vi "Interface tset.vi"() -> ()   [LabVIEW 2011]
uses:
  Criteria types.ctl
  Single criteria cluster.ctl
  Boolean operation.ctl
  Sequence steps config..ctl
  X-cont criteria/Criteria control.xctl
  Sequence step GUI.ctl
  X-cont Action select/Action select.xctl
  <vilib>/Utility/config.llb/NI_LVConfig.lvlib
panel:
  in  "Read":bool
  in  "Sequewnce jname":string="test"
  in  "Lagr":bool
  in  "Get":bool
  in  "Index":i32
  out "Array":string[](array[string])
  in  "Add":bool
  in  "Criteria 2":cluster{"Criteria":T1}(xcontrol)
  in  "Action select":cluster{"Action index":i32, "Data":dbl}(xcontrol)
  in  "Cluster 3":cluster{"Cluster 2":T3}
  out "Sequence step config":T5
  in  "Cluster":T3
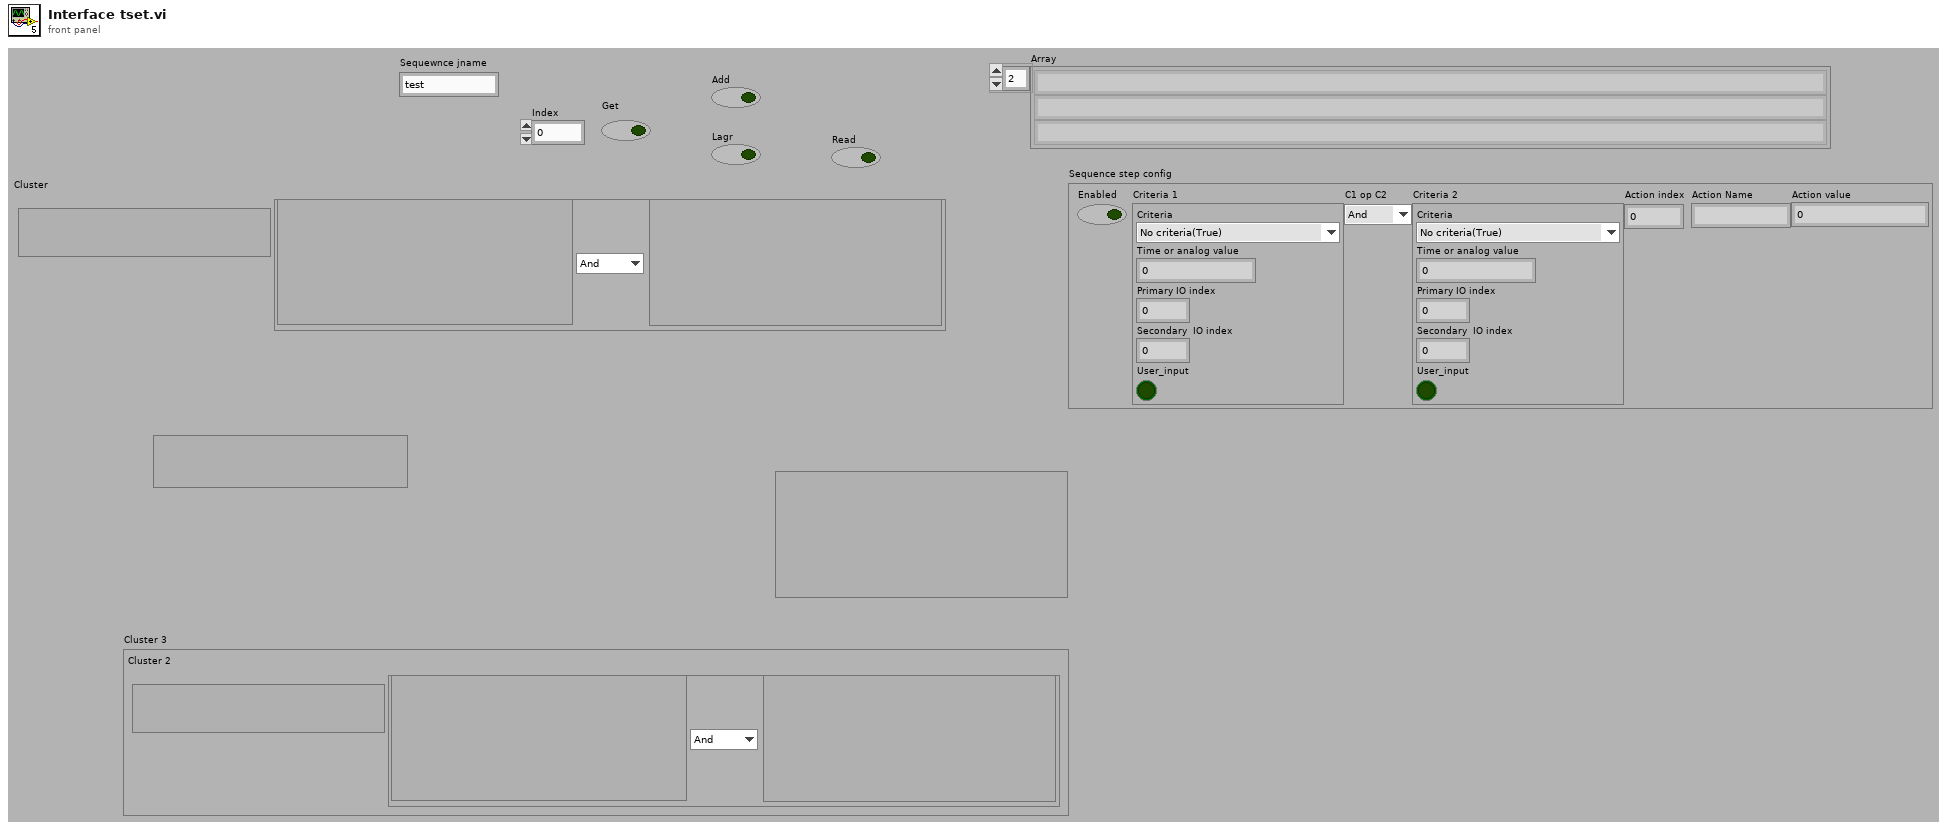
[diagram p1: front panel]
types:
  T1 = typedef "Single criteria cluster.ctl" = cluster{"Criteria":T2, "Time or analog value":dbl, "Primary IO index":i32, "Secondary  IO index":i32, "User_input":bool}
  T2 = typedef "Criteria types.ctl" = enum16{"No criteria(True)", "Time(s)", "Analog IO over", "Analog IO over or equal", "Analog IO under", "Analog IO under or equal", "Analog IO 1 minus Analog IO 2 over", "Digital IO True", "Digital IO False", "Operator approval"}
  T3 = typedef "Sequence step GUI.ctl" = cluster{"Action select":cluster{"Action index":i32, "Data":dbl}, "Criteria 1":cluster{"Criteria":T1}, "C1 op C2":T4, "Criteria 2":cluster{"Criteria":T1}}
  T4 = typedef "Boolean operation.ctl" = enum16{"And", "Or", "Xor", "Nand", "Nor", "Nxor", "Implies"}
  T5 = typedef "Sequence steps config..ctl" = cluster{"Enabled":bool, "Criteria 1":T1, "C1 op C2":T4, "Criteria 2":T1, "Action index":i32, "Action Name":string, "Action value":dbl}
  T6 = typedef "Action colleciton cluster.ctl" = cluster{"common":T7, "Action type":T9, "General command":T10, "PCP command":T11, "Tool command":T12}
  T7 = typedef "Action common elements.ctl" = cluster{"Name":string, "Adjuster type":T8, "Adjuster double default value":dbl}
  T8 = typedef "Action adjuster type.ctl" = enum16{"Non", "Double"}
  T9 = typedef "Action type.ctl" = enum16{"General", "PCP command", "Tool command"}
  T10 = typedef "General command list.ctl" = enum16{"No action"}
  T11 = typedef "PCP High Level Commands.ctl" = enum16{"HVPSU HV ON", "HVPSU HV OFF", "PCP PC", "PCP Local", "Update Motor Voltage", "Update Cable Resistance", "Final Motor Voltage", "Final Resistance"}
  T12 = typedef "Tool specific commands.ctl" = enum16{"controller relay 1 on", "controller relay 1 off", "controller relay 2 on", "controller relay 2 off", "Solonoid 1 (master) on", "Solonoid 1 (master) off", "Solonoid 2 (Stroker) on", "Solonoid 2 (Stroker) off", "Solonoid 3 (Anchor) on", "Solonoid 3 (Anchor) off", "Controller relay 1 & 2 on", "Controller relay 1 & 2 off", "Controller relay 1 on, 2 off", "Controller relay 1 off, 2 on", "STROKER tool: Stop Force Mon", "High-G Stop", "High-G Get data", "High-G Stop Get data", "STROKER tool: Stroke out", "STROKER tool: Stroke in", "STROKER tool: Stroke stop", "STROKER tool: Stroke go to", "STROKER tool: Stop Homing", "STROKER tool: Start Force Mon dir in", "STROKER tool: Start Force Mon dir out", "Controller STOP"}
  T13 = typedef "Fixed Analog Channel Definition.ctl" = cluster{"ID":u16, "Name":string, "Quantity":T14, "Unit":string, "Maximum upd":T15, "Comment":string, "Help file Name":string, "Help file Section ":string, "Category":T16, "User adjustable Scaling":bool, "Default Scaling":T17, "In use":bool, "Default Unit":i32}
  T14 = typedef "Quantity enum.ctl" = enum16{"Acceleration", "Angle", "Current", "Force", "Distance", "Pressure", "Resistance", "Rotational Speed", "Speed", "Temperature", "Tension", "Torque", "Voltage", "Weight"}
  T15 = typedef "Update frequensies.ctl" = enum16{"2 Hz", "1 Hz", "0.1 Hz"}
  T16 = typedef "Channel catagory Enum.ctl" = enum16{"No Category", "Power", "Temperature", "Pressure"}
  T17 = typedef "Scaling.ctl" = cluster{"Gain":dbl, "Offset":dbl}
  T18 = typedef "Fixed Digital Channel Definition.ctl" = cluster{"ID":u16, "Name":string, "NA Text":string, "Off Text":string, "On Text":string, "Maximum upd":T15, "Comment":string, "Help file Name":string, "Help file Section ":string, "Catagory":T16, "In use":bool}
  T19 = typedef "NI_LVConfig.lvlib/Config Data RefNum.ctl" = refnum<k1>
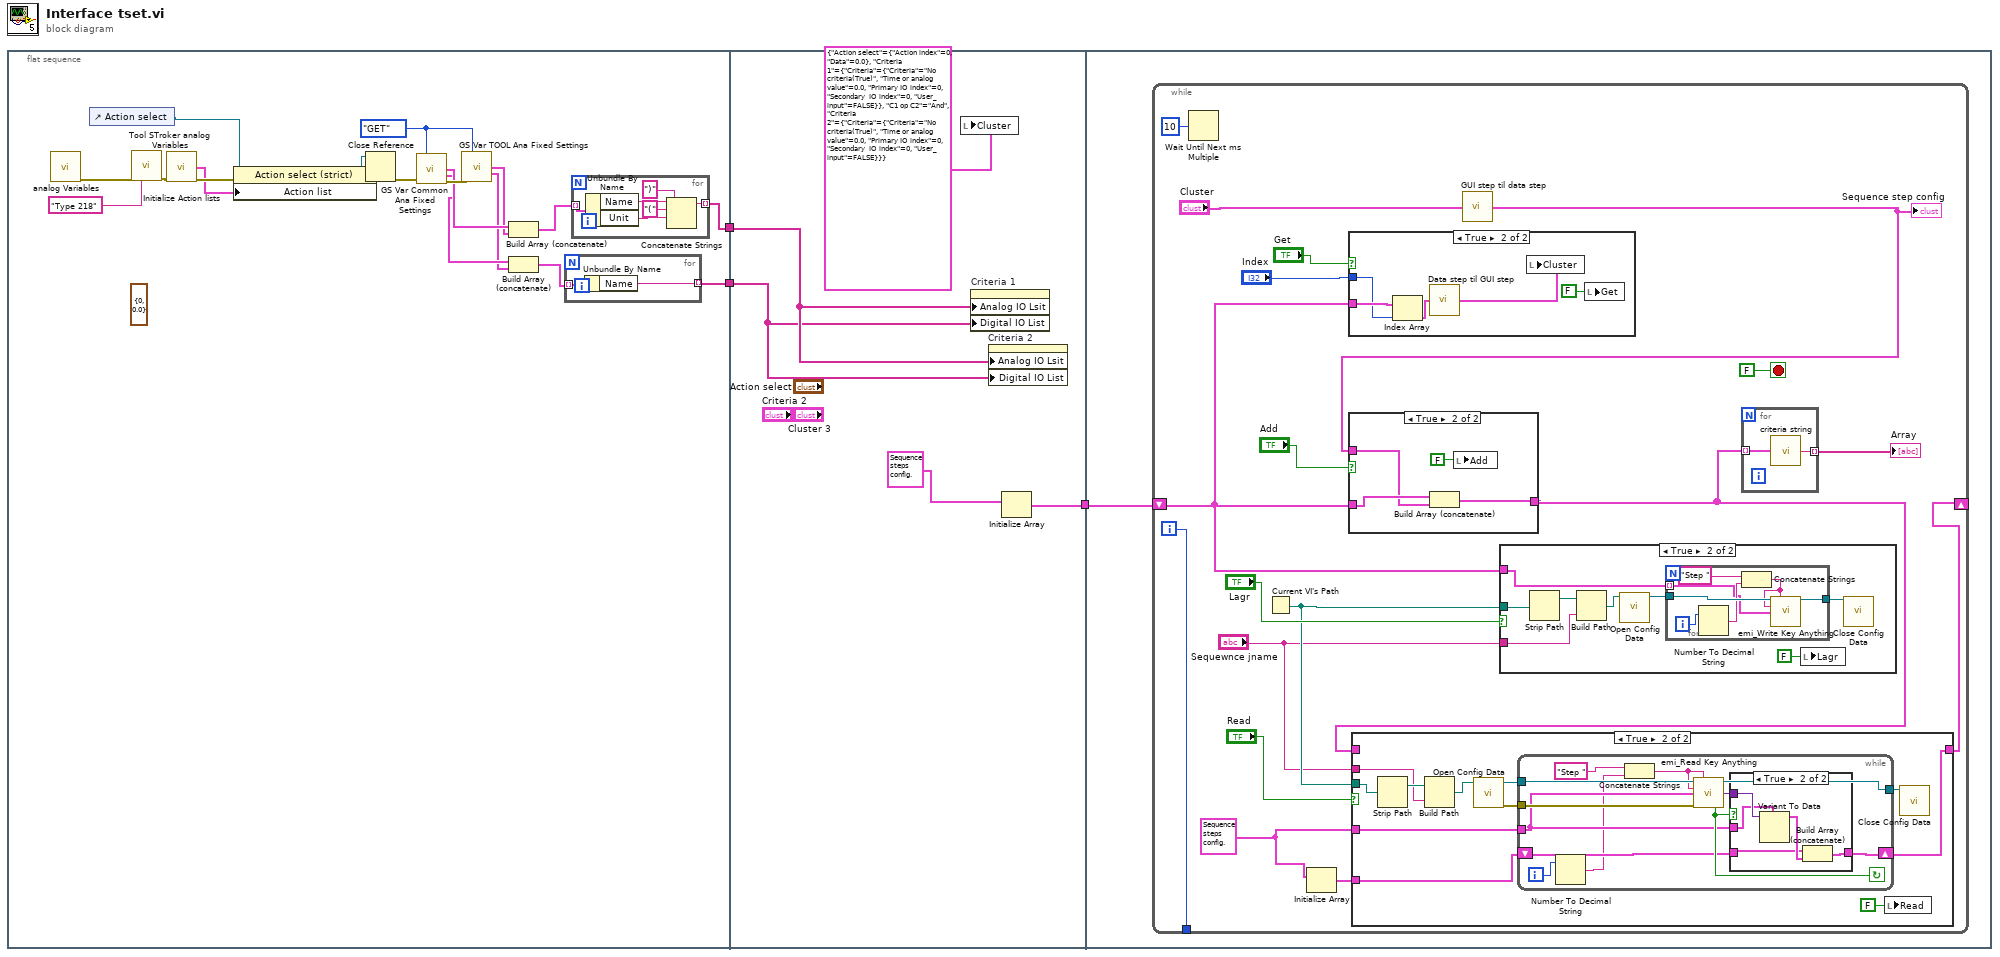
[diagram p0: block diagram]
diagram:
  n1 = flat-sequence {
    tunnel: [w7] -> w3
    tunnel: [w6] -> w2
    tunnel: w3 -> [w35]
    tunnel: w2 -> [w34]
    tunnel: [w31] -> w1
    tunnel: w1 -> [w36]
    frame #0 {
      (unwired) cluster{"Action index":i32, "Data":dbl} {"Action index"=0, "Data"=0.0} ("Action select")
      w14 = enum16{"GET", "SET"}."GET" ("Action(GET)")
      n2 = call "analog Variables.vi"() -> ("error out"=w19:errorcluster)  [unwired: 15 in]
      n3 = control-ref of="Action select"() -> (w5:refnum<vi>)
      n4 = call "Tool STroker analog Variables.vi"("error in (no error)"=w19, "Tool folder name"="Type 218") -> ("error out"=w18:errorcluster)  [unwired: 13 in]
      n5 = call "Initialize Action lists.vi"("error in (no error)"=w18) -> ("Actions"=w4:T6[], "error out"=w20:errorcluster)  [unwired: 12 in, 1 out]
      n6 = property class="Action select (strict)"(reference=w5, error in=w20, "Action list"=w4) -> (reference out=w22:refnum<vi>, error out=w21:errorcluster)
      n7 = Close Reference(reference=w22, error in (no error)=w21) -> (error out=w16:errorcluster)
      n8 = call "GS Var Common Ana Fixed Settings.vi"("Action(GET)"=w14, "error in (no error)"=w16) -> ("Common Analog Var Fixed out"=w13:T13[], "Common Digital var Fixed"=w11:T18[], "error out"=w15:errorcluster)  [unwired: 11 in]
      n9 = call "GS Var TOOL Ana Fixed Settings.vi"("Action(GET)"=w14, "error in (no error)"=w15) -> ("Tool Analog var Fixed out"=w12:T13[], "Tool Digital Var Fixed out"=w10:T18[])  [unwired: 11 in, 1 out]
      n10 = Build Array (concatenate)(w13, w12) -> (w9:T13[])
      n11 = Build Array (concatenate)(w11, w10) -> (w8:T18[])
      n12 = for {
        tunnel: w8 -> [w24] mode=indexing
        tunnel: [w23] -> w6 mode=indexing
        n13 = Unbundle By Name(w24) -> ("Name"=w23:string)
      }
      n14 = for {
        tunnel: w9 -> [w30] mode=indexing
        tunnel: [w28] -> w7 mode=indexing
        n15 = Unbundle By Name(w30) -> ("Name"=w29:string, "Unit"=w27:string)
        n16 = Concatenate Strings(w29, "(" ("string"), w27, ")" ("string")) -> (w28:string)
      }
    }
    frame #1 {
      n17 = local write "Cluster"(T3 {"Action select"={"Action index"=0, "Data"=0.0}, "Criteria 1"={"Criteria"={"Criteria"=enum."No criteria(True)", "Time or analog value"=0.0, "Primary IO index"=0, "Secondary  IO index"=0, "User_input"=FALSE}}, "C1 op C2"=enum."And", "Criteria 2"={"Criteria"={"Criteria"=enum."No criteria(True)", "Time or analog value"=0.0, "Primary IO index"=0, "Secondary  IO index"=0, "User_input"=FALSE}}} ("Cluster")) -> ()
      n18 = property on="Criteria 1" class="Criteria control (strict)"("Analog IO Lsit"=w35, "Digital IO List"=w34) -> ()  [unwired: 2 in, 2 out]
      n19 = property on="Criteria 2" class="Criteria control (strict)"("Analog IO Lsit"=w35, "Digital IO List"=w34) -> ()  [unwired: 2 in, 2 out]
      n20 = Initialize Array(T5 {"Enabled"=FALSE, "Criteria 1"={"Criteria"=enum."No criteria(True)", "Time or analog value"=0.0, "Primary IO index"=0, "Secondary  IO index"=0, "User_input"=FALSE}, "C1 op C2"=enum."And", "Criteria 2"={"Criteria"=enum."No criteria(True)", "Time or analog value"=0.0, "Primary IO index"=0, "Secondary  IO index"=0, "User_input"=FALSE}, "Action index"=0, "Action Name"="", "Action value"=0.0} ("Sequence step config")) -> (w31:T5[])  [unwired: 1 in]
    }
    frame #2 {
      n21 = while {
        shift-right: [w37] -> _
        shift-left: w36 -> [w45]
        tunnel: [w46] -> _
        i -> [w46]
        stop <- FALSE stop-if-true
        w40 = T5 {"Enabled"=FALSE, "Criteria 1"={"Criteria"=enum."No criteria(True)", "Time or analog value"=0.0, "Primary IO index"=0, "Secondary  IO index"=0, "User_input"=FALSE}, "C1 op C2"=enum."And", "Criteria 2"={"Criteria"=enum."No criteria(True)", "Time or analog value"=0.0, "Primary IO index"=0, "Secondary  IO index"=0, "User_input"=FALSE}, "Action index"=0, "Action Name"="", "Action value"=0.0} ("data step cluster")
        n22 = Wait Until Next ms Multiple(millisecond multiple=u32 10) -> ()  [unwired: 1 out]
        n23 = Current VI's Path() -> (path=w42:path)
        n24 = Initialize Array(w40) -> (w39:T5[])  [unwired: 1 in]
        n25 = case shown="True" "Get" {
          tunnel: "Index" -> [_ w102]
          tunnel: w45 -> [_ w103]
          frame False {
          }
          frame True {
            n26 = Index Array(array=w103, index=w102) -> (element=w101:T5)
            n27 = call "Data step til GUI step.vi"("data step cluster"=w101) -> ("GUI step clluster"=w100:T3)  [unwired: 13 in, 1 out]
            n28 = local write "Cluster"(w100) -> ()
            n29 = local write "Get"(FALSE ("Get")) -> ()
          }
        }
        n30 = call "GUI step til data step.vi"("GUI step clluster"="Cluster") -> ("data step cluster"=w50:T5)  [unwired: 14 in]
        "Sequence step config" <- w50
        n31 = case shown="True" "Add" {
          tunnel: w45 -> [w107 w110]
          tunnel: [w107 w109] -> w38
          tunnel: w50 -> [_ w108]
          frame False {
          }
          frame True {
            n32 = Build Array (concatenate)(w110, w108) -> (w109:T5[])
            n33 = local write "Add"(FALSE ("Add")) -> ()
          }
        }
        n34 = case shown="True" "Read" {
          tunnel: w42 -> [_ w64]
          tunnel: "Sequewnce jname" -> [_ w63]
          tunnel: w40 -> [_ w59]
          tunnel: w39 -> [_ w58]
          tunnel: w38 -> [w55 _]
          tunnel: [w55 w56] -> w37
          frame False {
          }
          frame True {
            n35 = Strip Path(path=w64) -> (stripped path=w65:path)  [unwired: 1 out]
            n36 = Build Path(base path=w65, name or relative path=w63) -> (appended path=w62:path)
            n37 = call <vilib>:"Open Config Data.vi"("configuration file path"=w62) -> ("error out"=w60:errorcluster, "refnum"=w61:T19)  [unwired: 8 in, 1 out]
            n38 = while {
              tunnel: w61 -> [w71]
              tunnel: w60 -> [w78]
              tunnel: w59 -> [w73]
              shift-right: [w76] -> w56
              shift-left: w58 -> [w75]
              tunnel: [w72] -> w57
              i -> [w70]
              stop <- w77 continue-if-true
              n39 = Number To Decimal String(number=w70) -> (decimal integer string=w69:string)  [unwired: 1 in]
              n40 = Concatenate Strings("Step " ("Section(Default)"), w69) -> (w67:string)
              n41 = call "emi_Read Key Anything.vi"("Ini file refnum"=w71, "Section(Default)"=w67, "Name"=w67, "Anything"=w73, "error in (no error)"=w78) -> ("Ini file refnum out"=w72:T19, "Anything Out"=w74:variant, "Found"=w77:bool)  [unwired: 7 in, 1 out]
              n42 = case shown="True" w77 {
                tunnel: [w79 w81] -> w76
                tunnel: w75 -> [w79 w80]
                tunnel: w74 -> [_ w84]
                tunnel: w73 -> [_ w83]
                frame False {
                }
                frame True {
                  n43 = Variant To Data(type=w83, Variant=w84) -> (data=w82:T5)  [unwired: 1 in, 1 out]
                  n44 = Build Array (concatenate)(w80, w82) -> (w81:T5[])
                }
              }
            }
            n45 = local write "Read"(FALSE ("Read")) -> ()
            n46 = call <vilib>:"Close Config Data.vi"("refnum"=w57) -> ()  [unwired: 9 in, 2 out]
          }
        }
        n47 = case shown="True" "Lagr" {
          tunnel: w45 -> [_ w86]
          tunnel: "Sequewnce jname" -> [_ w89]
          tunnel: w42 -> [_ w91]
          frame False {
          }
          frame True {
            n48 = Strip Path(path=w91) -> (stripped path=w90:path)  [unwired: 1 out]
            n49 = Build Path(base path=w90, name or relative path=w89) -> (appended path=w88:path)
            n50 = call <vilib>:"Open Config Data.vi"("configuration file path"=w88) -> ("refnum"=w87:T19)  [unwired: 8 in, 2 out]
            n51 = for {
              tunnel: w87 -> [w99]
              tunnel: w86 -> [w94] mode=indexing
              tunnel: [w93] -> w85
              i -> [w97]
              n52 = Number To Decimal String(number=w97) -> (decimal integer string=w96:string)  [unwired: 1 in]
              n53 = Concatenate Strings("Step " ("Section(Default)"), w96) -> (w95:string)
              n54 = call "emi_Write Key Anything.vi"("Ini file refnum"=w99, "Section(Default)"=w95, "Name"=w95, "Anything"=w94) -> ("Ini file refnum out"=w93:T19)  [unwired: 10 in, 1 out]
            }
            n55 = local write "Lagr"(FALSE ("Lagr")) -> ()
            n56 = call <vilib>:"Close Config Data.vi"("refnum"=w85) -> ()  [unwired: 9 in, 2 out]
          }
        }
        n57 = for {
          tunnel: w38 -> [w106] mode=indexing
          tunnel: [w105] -> w49 mode=indexing
          n58 = call "criteria string.vi"("Sequence step config"=w106) -> ("Full criteria string"=w105:string)  [unwired: 13 in, 1 out]
        }
        "Array" <- w49
      }
    }
  }
